vi "Init.vi"(8 "Error In":errorcluster, 10 "IConfigure":refnum<class "IConfigure.lvclass">, 11 "object in":refnum<class "PXI-5441.lvclass">) -> (0 "Error Out":errorcluster, 3 "object out":refnum<class "PXI-5441.lvclass">)   [LabVIEW 2023, in "PXI-5441.lvlib" / "PXI-5441.lvclass"]
uses:
  PXI-5441.lvclass
  PXI-5441.lvclass/PXI-5441.ctl
  IConfigureViaSessionHandle_interface/IConfigure NI-FGEN.lvclass
  IConfigure_interface/IConfigure.lvclass
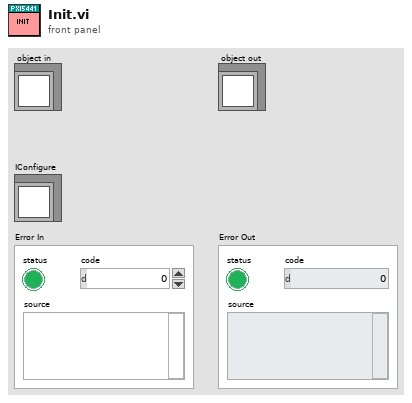
[diagram p1: front panel]
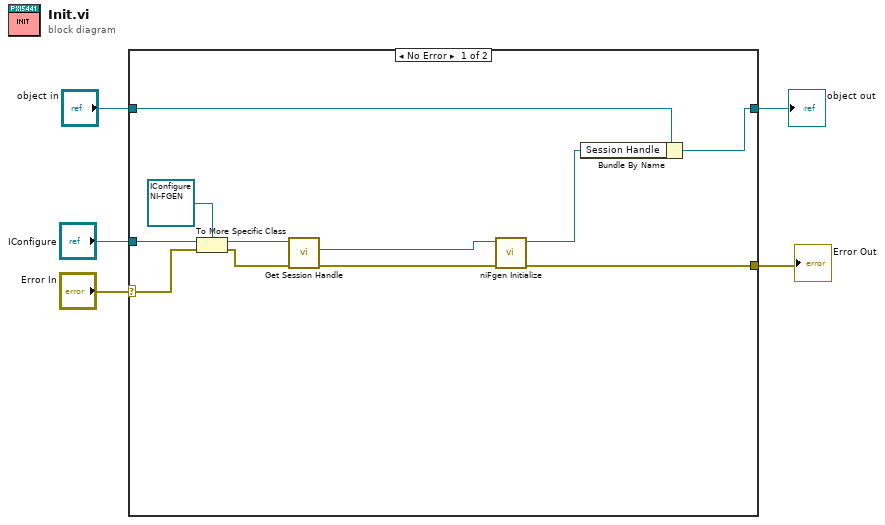
[diagram p0: block diagram]
diagram:
  n1 = case shown="No Error" "Error In" {
    selector: "Error In" -> [w15 w18]
    tunnel: [w11 w18] -> w4
    tunnel: [w8 w17] -> w2
    tunnel: "object in" -> [w9 w17]
    tunnel: "IConfigure" -> [w16 _]
    frame No Error {
      n2 = To More Specific Class(target class=refnum<class "IConfigure NI-FGEN.lvclass"> refnum ("HAL.lvlib:IConfigureViaSessionHandle"), reference=w16, error in=w15) -> (specific class reference=w13:refnum<class "IConfigure NI-FGEN.lvclass">, error out=w14:errorcluster)
      n3 = call-dynamic "Get Session Handle.vi"("Error In"=w14, "object in"=w13) -> ("Error Out"=w12:errorcluster, "Session Handle"=w10:refnum<k15>)  [unwired: 7 in, 1 out]
      n4 = call <instrlib>:"niFgen Initialize.vi"("error in (no error)"=w12, "Resource Name"=w10) -> ("error out"=w11:errorcluster, "Instrument Handle Out"=w7:refnum<k15>)  [unwired: 8 in]
      n5 = Bundle By Name(cluster=w9, "Session Handle"=w7) -> (w8:refnum<class "PXI-5441.lvclass">)
    }
    frame Error {
    }
  }
  "Error Out" <- w4
  "object out" <- w2
